vi "2012_12_29 Durability8 Main.vi"() -> ()   [LabVIEW 2011]
uses:
  MotorTypeDef.ctl
  <vilib>/DAQmx/write.llb/DAQmx Write (Counter Time 1Chan 1Samp).vi
  <vilib>/DAQmx/read.llb/DAQmx Read (Analog 1D Wfm NChan NSamp).vi
  <vilib>/Utility/TradDaqScaling.llb/Convert Thermistor Reading (waveform).vi
  <vilib>/DAQmx/miscellaneous.llb/DAQmx Fill In Error Info.vi
  <vilib>/measure/madcrms.llb/Averaged DC-RMS for N Chan.vi
  <vilib>/measure/madcrms.llb/Basic Averaged DC-RMS for 1 Chan.vi
  <vilib>/measure/matone.llb/Extract Single Tone Information 1 Chan.vi
  <vilib>/express/express arith-compare/Formula/XNode/ExpressFormulaBlockNode.xnode
  <vilib>/measure/NI_MAPro.lvlib
panel:
  out "for loop":i32
  out "Saving Data":bool
  in  "Coarse File Path":path=path "Durability/coarse.lvm"
  in  "Fine File Path":path=path "Durability/fine.lvm"
  out "Voltages":waveform(dbl)[](graph)
  out "Currents":waveform(dbl)[](graph)
  out "RMS Voltages 2":waveform(dbl)(graph)
  in  "Motor 8":T1 {"Efficiency" format="%#_3g%%"; "Supply Voltage (V)" format="%#_3f"; "Power Output (W)" format="%#_3g"; "Power Usage (W)" format="%#_3g"; "Torque (mNm)" format="%#_3g"; "RPM" scale=0.0..40000.0 scale format="%#.6p"}
  in  "Motor 7":T1 {"Efficiency" format="%#_3g%%"; "Supply Voltage (V)" format="%#_3f"; "Power Output (W)" format="%#_3g"; "Power Usage (W)" format="%#_3g"; "Torque (mNm)" format="%#_3g"; "RPM" scale=0.0..40000.0 scale format="%#.6p"}
  in  "Motor 6":T1 {"Efficiency" format="%#_3g%%"; "Supply Voltage (V)" format="%#_3f"; "Power Output (W)" format="%#_3g"; "Power Usage (W)" format="%#_3g"; "Torque (mNm)" format="%#_3g"; "RPM" scale=0.0..40000.0 scale format="%#.6p"}
  in  "Motor 5":T1 {"Efficiency" format="%#_3g%%"; "Supply Voltage (V)" format="%#_3f"; "Power Output (W)" format="%#_3g"; "Power Usage (W)" format="%#_3g"; "Torque (mNm)" format="%#_3g"; "RPM" scale=0.0..40000.0 scale format="%#.6p"}
  in  "Motor 4":T1 {"Efficiency" format="%#_3g%%"; "Supply Voltage (V)" format="%#_3f"; "Power Output (W)" format="%#_3g"; "Power Usage (W)" format="%#_3g"; "Torque (mNm)" format="%#_3g"; "RPM" scale=0.0..40000.0 scale format="%#.6p"}
  in  "Motor 3":T1 {"Efficiency" format="%#_3g%%"; "Supply Voltage (V)" format="%#_3f"; "Power Output (W)" format="%#_3g"; "Power Usage (W)" format="%#_3g"; "Torque (mNm)" format="%#_3g"; "RPM" scale=0.0..40000.0 scale format="%#.6p"}
  in  "Motor 2":T1 {"Efficiency" format="%#_3g%%"; "Supply Voltage (V)" format="%#_3f"; "Power Output (W)" format="%#_3g"; "Power Usage (W)" format="%#_3g"; "Torque (mNm)" format="%#_3g"; "RPM" scale=0.0..40000.0 scale format="%#.6p"}
  in  "Motor 1":T1 {"Efficiency" format="%#_3g%%"; "Supply Voltage (V)" format="%#_3f"; "Power Output (W)" format="%#_3g"; "Power Usage (W)" format="%#_3g"; "Torque (mNm)" format="%#_3g"; "RPM" scale=0.0..40000.0 scale format="%#.6p"}
  out "Motor Temp":dbl(slide) scale=90.0..110.0
  out "Tank Temp":dbl(slide) scale=90.0..110.0
  out "RMS Voltages":waveform(dbl)[](graph)
  out "RMS Currents":waveform(dbl)[](graph)
  in  "Temp Probe\nOn Motor":dbl=1.0
  out "loop time (ms)":u32
  in  "stop":bool
  in  "Unlock PWM":bool=TRUE
  in  "PWM 2":dbl(slide)=100.0 min=0.0 max=100.0 step=5.0 scale=0.0..100.0
  in  "PWM 1":dbl(slide) min=0.0 max=100.0 step=5.0 scale=0.0..100.0
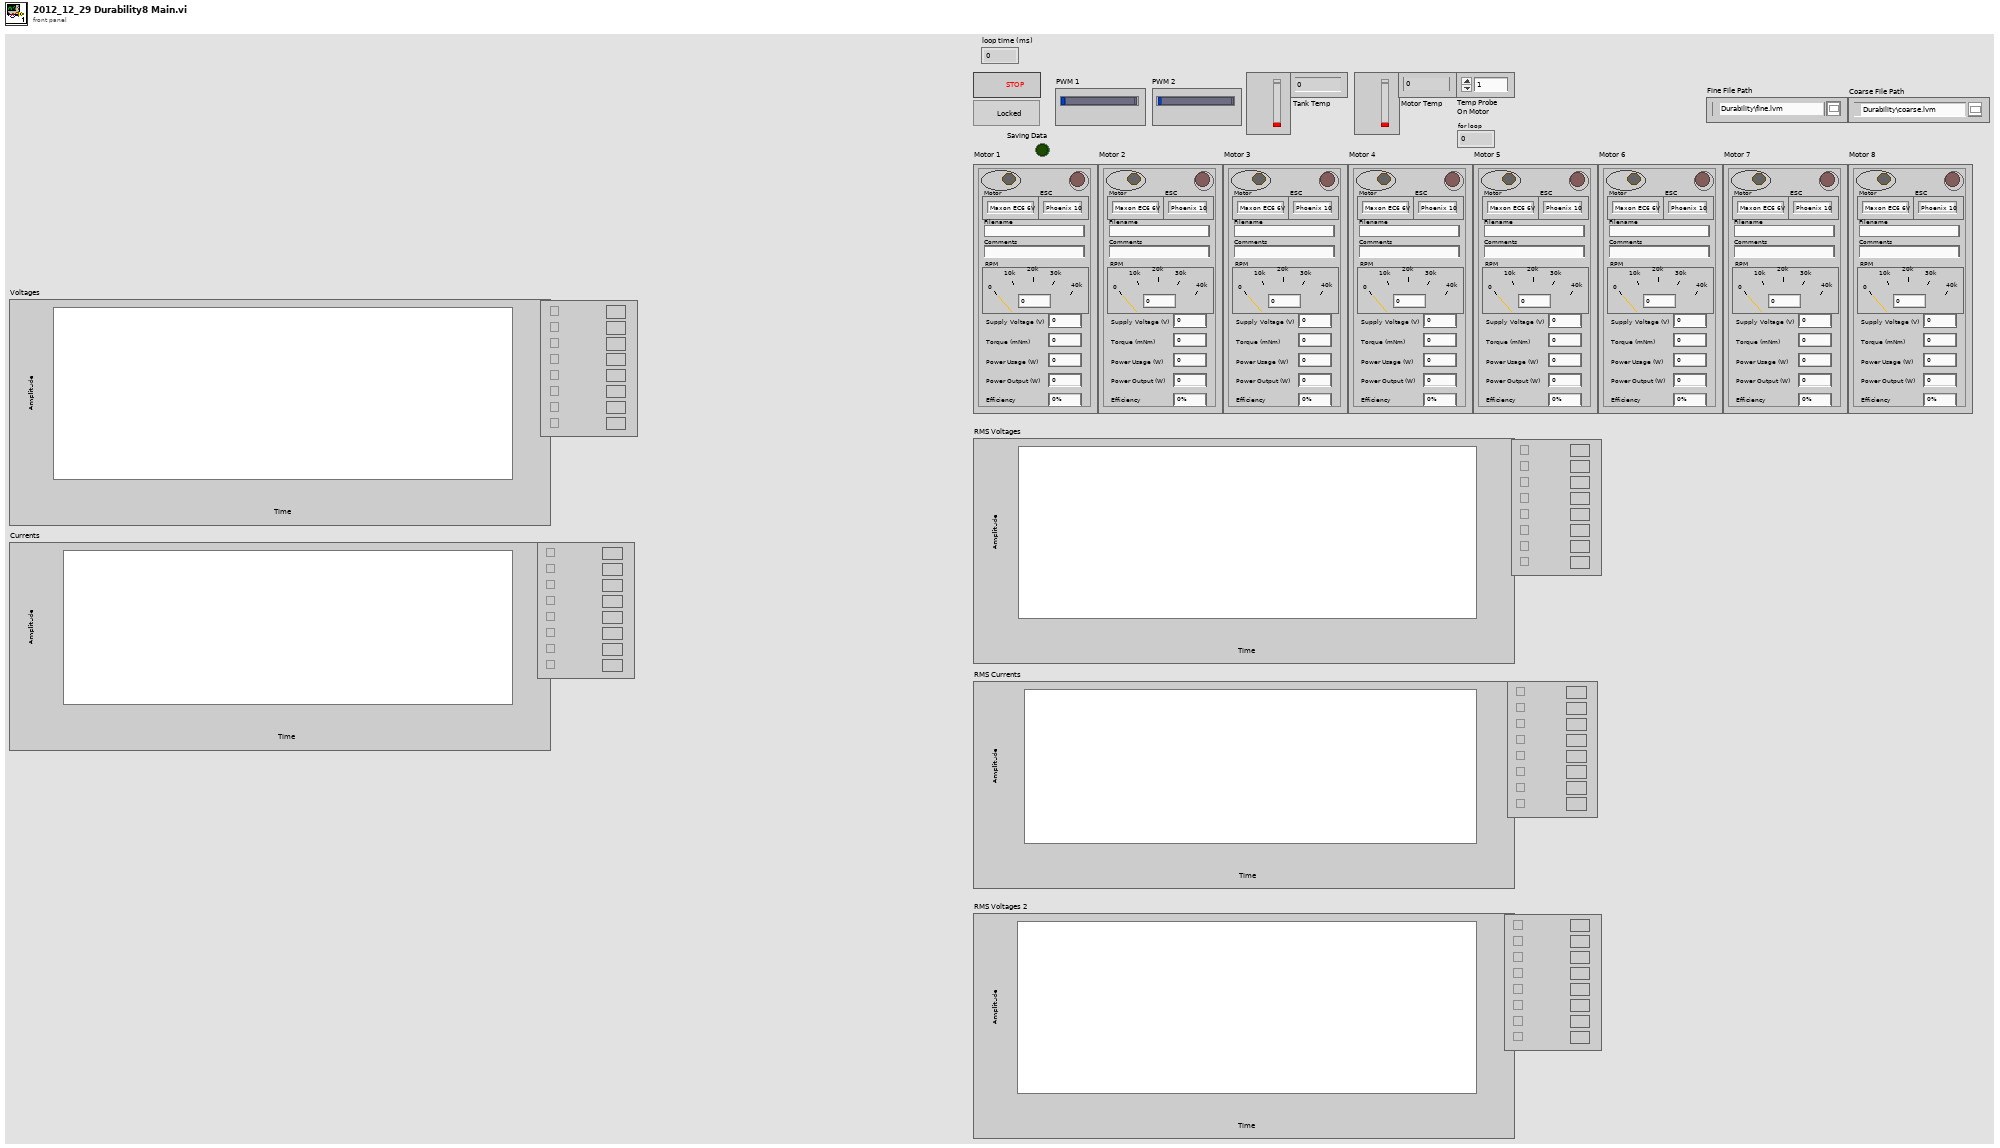
[diagram p1: front panel]
types:
  T1 = typedef "MotorTypeDef.ctl" = cluster{"Enabled":bool, "Fail":bool, "RPM":dbl, "Motor":enum16{"Maxon EC6 6V", "Maxon EC4 6V", "FH 0620 6V", "FH 0620 12V"}, "ESC":enum16{"Phoenix 10", "Maxon", "FH 1801"}, "Torque (mNm)":dbl, "Power Usage (W)":dbl, "Power Output (W)":dbl, "Supply Voltage (V)":dbl, "Efficiency":dbl, "Filename":string, "Comments":string}
  T2 = enum8{"Enabled", "Disabled", "Disabled and Grayed Out"}
  T3 = enum16{"Maxon EC6 6V", "Maxon EC4 6V", "FH 0620 6V", "FH 0620 12V"}
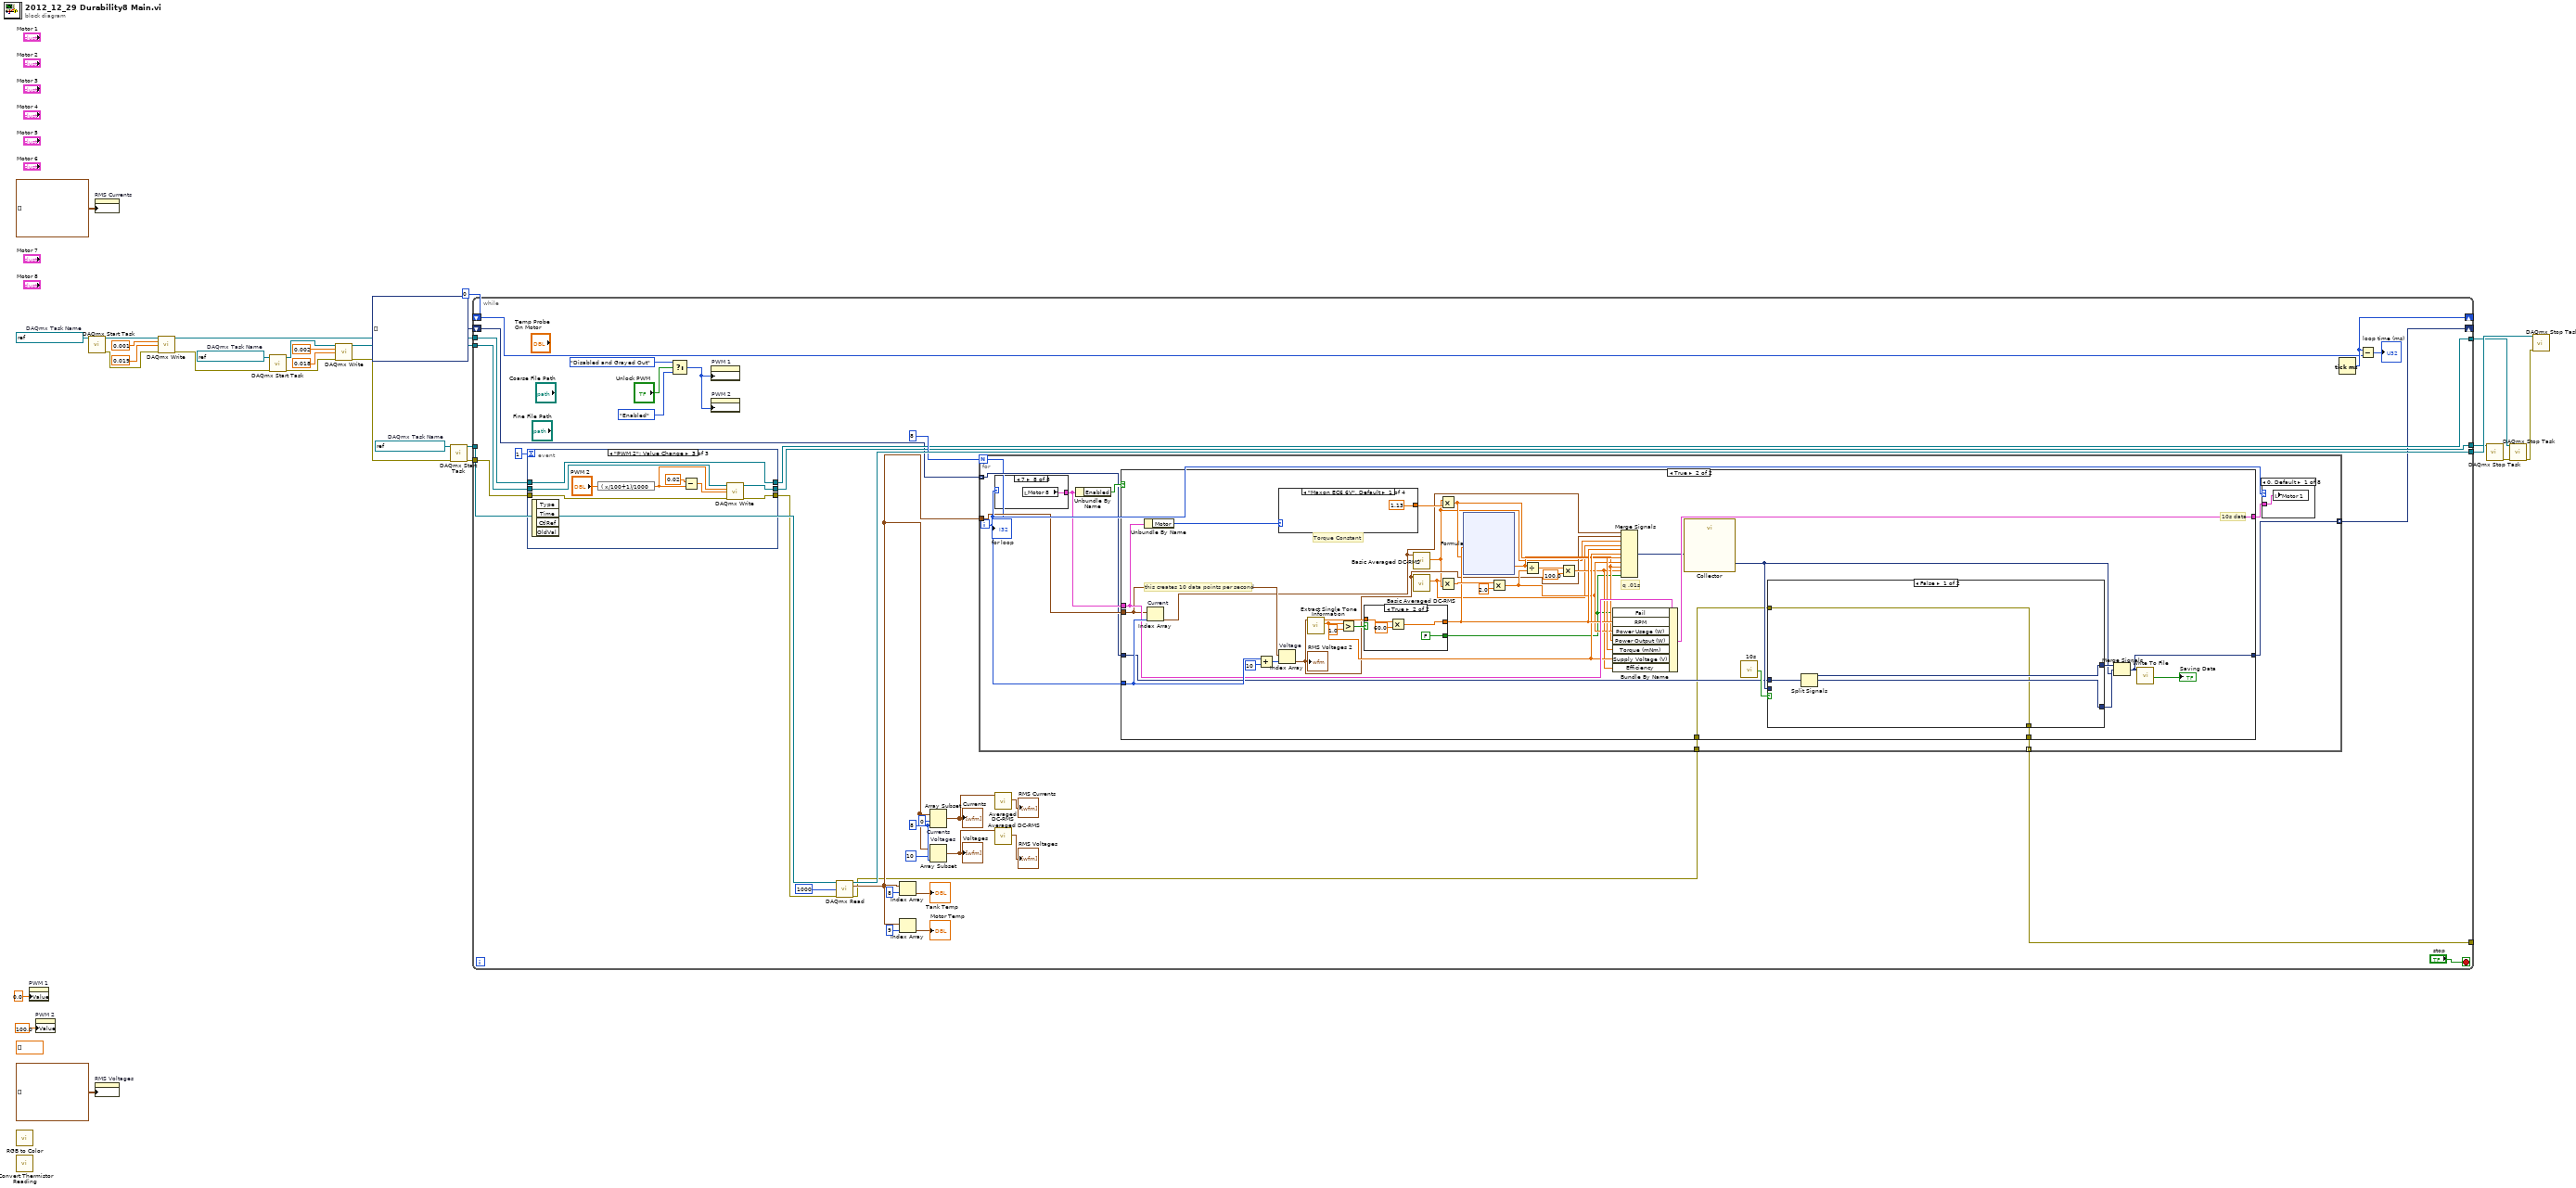
[diagram p0: block diagram]
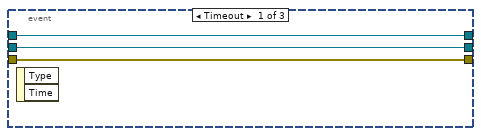
[diagram p2: hidden frame]
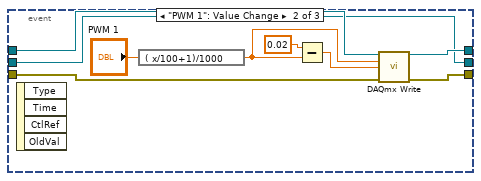
[diagram p3: hidden frame]
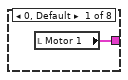
[diagram p4: hidden frame]
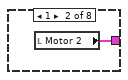
[diagram p5: hidden frame]
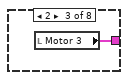
[diagram p6: hidden frame]
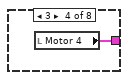
[diagram p7: hidden frame]
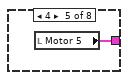
[diagram p8: hidden frame]
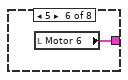
[diagram p9: hidden frame]
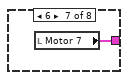
[diagram p10: hidden frame]
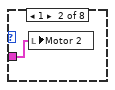
[diagram p11: hidden frame]
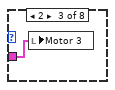
[diagram p12: hidden frame]
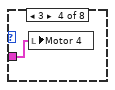
[diagram p13: hidden frame]
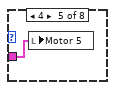
[diagram p14: hidden frame]
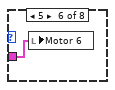
[diagram p15: hidden frame]
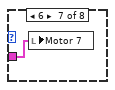
[diagram p16: hidden frame]
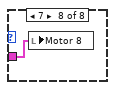
[diagram p17: hidden frame]
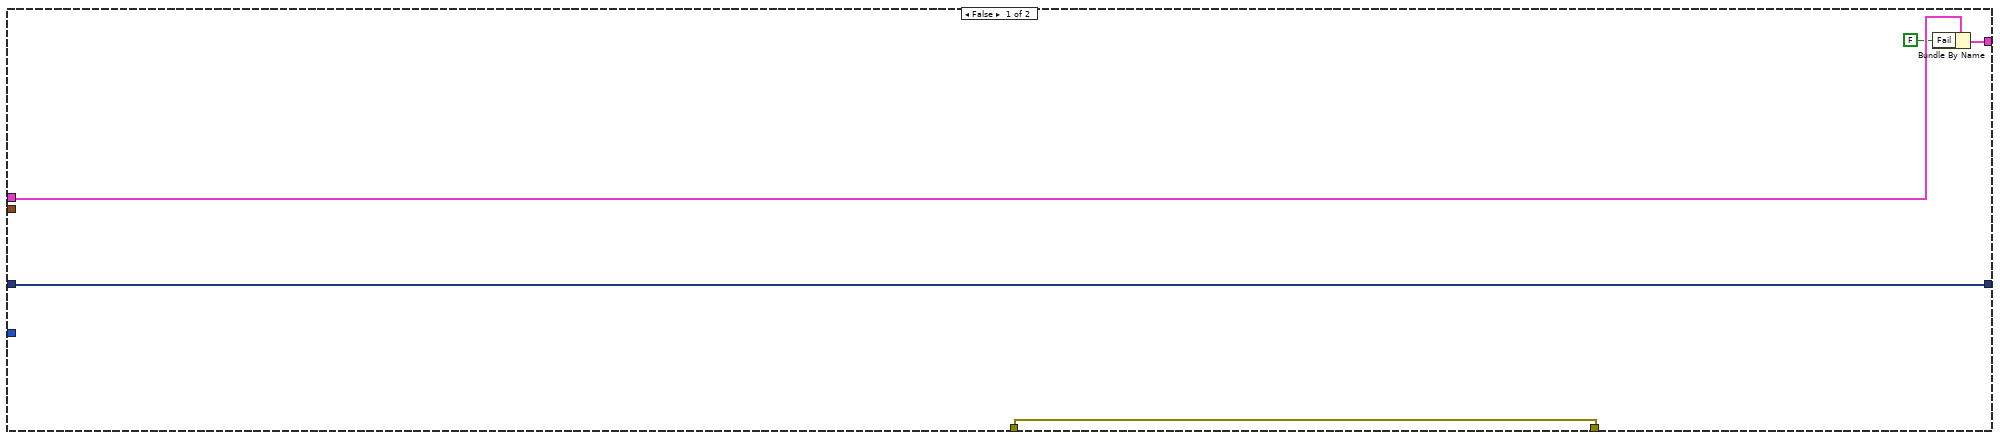
[diagram p18: hidden frame]
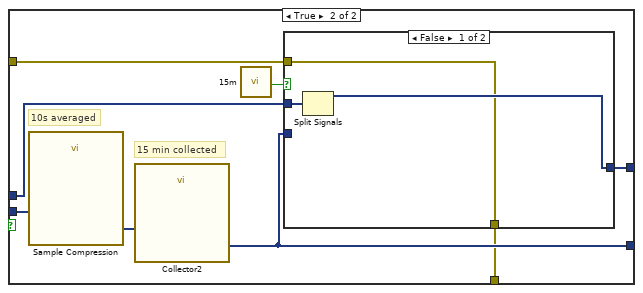
[diagram p19: hidden frame]
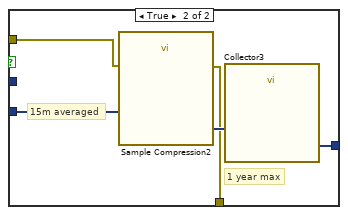
[diagram p20: hidden frame]
diagram:
  (unwired) dbl[] [] ("History Data")
  w23 = refnum<k21> "Durability8 PWM2"  # DAQmx Task Name
  w24 = refnum<k21> "Durability8 PWM1"  # DAQmx Task Name
  w28 = refnum<k21> "Durability8 Acquire"  # DAQmx Task Name
  n1 = call <vilib>:"RGB to Color.vi"() -> ()  [unwired: 3 in, 1 out]
  n2 = call-poly <vilib>:"Convert Thermistor Reading.vi"() -> ()  [unwired: 7 in, 1 out]
  n3 = property on="PWM 1" class="Slide (strict)"("Value"=0.0 ("PWM 1")) -> ()  [unwired: 2 in, 2 out]
  n4 = property on="PWM 2" class="Slide (strict)"("Value"=100.0 ("PWM 2")) -> ()  [unwired: 2 in, 2 out]
  n5 = call <vilib>:"DAQmx Start Task.vi"("task/channels in"=w24) -> ("task out"=w20:refnum<k21>, "error out"=w18:errorcluster)  [unwired: 13 in]
  n6 = property on="RMS Currents" class="WFChart (strict)"("History Data"=waveform(dbl)[][] []) -> ()  [unwired: 2 in, 2 out]
  n7 = property on="RMS Voltages" class="WFChart (strict)"("History Data"=waveform(dbl)[][] []) -> ()  [unwired: 2 in, 2 out]
  n8 = call-poly <vilib>:"DAQmx Write.vi"("task/channels in"=w20, "high time"=0.001 ("data"), "low time"=0.019 ("data"), "error in"=w18) -> ("task out"=w22:refnum<k21>, "error out"=w17:errorcluster)  [unwired: 9 in, 1 out]
  n9 = call <vilib>:"DAQmx Start Task.vi"("task/channels in"=w23, "error in"=w17) -> ("task out"=w19:refnum<k21>, "error out"=w16:errorcluster)  [unwired: 12 in]
  n10 = call-poly <vilib>:"DAQmx Write.vi"("task/channels in"=w19, "high time"=0.002 ("data"), "low time"=0.018 ("data"), "error in"=w16) -> ("task out"=w21:refnum<k21>, "error out"=w15:errorcluster)  [unwired: 9 in, 1 out]
  n11 = call <vilib>:"DAQmx Start Task.vi"("task/channels in"=w28, "error in"=w15) -> ("task out"=w27:refnum<k21>, "error out"=w25:errorcluster)  [unwired: 12 in]
  n12 = while {
    tunnel: w27 -> [w63]
    tunnel: [w62] -> w26
    tunnel: w25 -> [w39]
    tunnel: [w29] -> _
    shift-right: [w56] -> _
    shift-left: u32 0 ("millisecond timer value") -> [w55]
    tunnel: w22 -> [w41]
    tunnel: w21 -> [w40]
    tunnel: [w38] -> w14
    tunnel: [w37] -> w5
    shift-right: [w32] -> _
    shift-left: dynamicdata[] [] -> [w31]
    stop <- "stop" stop-if-true
    w51 = 8 ("length")
    n13 = event shown="[2] \"PWM 2\": Value Change" {
      selector: _ -> [_ _ _]
      dyn-events: _ -> [_ _ _]
      timeout: 1 -> [_ _ _]
      tunnel: w41 -> [w66 w71 w77]
      tunnel: w40 -> [w65 w69 w76]
      tunnel: [w66 w70 w77] -> w38
      tunnel: [w65 w69 w78] -> w37
      tunnel: [w64 w68 w79] -> w33
      tunnel: w39 -> [w64 w67 w80]
      event Timeout {
        n14 = event-data() -> ()  [unwired: 1 in, 2 out]
      }
      event "PWM 1": Value Change {
        n15 = event-data() -> ()  [unwired: 1 in, 4 out]
        n16 = expression code="( x/100+1)/1000"("PWM 1") -> (w72:dbl)
        n17 = Subtract(x=0.02 ("y"), y=w72) -> (x-y=w73:dbl)
        n18 = call-poly <vilib>:"DAQmx Write.vi"("task/channels in"=w71, "high time"=w72, "low time"=w73, "error in"=w67) -> ("task out"=w70:refnum<k21>, "error out"=w68:errorcluster)  [unwired: 9 in, 1 out]
      }
      event "PWM 2": Value Change {
        n19 = event-data() -> ()  [unwired: 1 in, 4 out]
        n20 = expression code="( x/100+1)/1000"("PWM 2") -> (w84:dbl)
        n21 = Subtract(x=0.02, y=w84) -> (x-y=w82:dbl)
        n22 = call-poly <vilib>:"DAQmx Write.vi"("task/channels in"=w76, "high time"=w84, "low time"=w82, "error in"=w80) -> ("task out"=w78:refnum<k21>, "error out"=w79:errorcluster)  [unwired: 9 in, 1 out]
      }
    }
    n23 = Select(t=T2."Disabled and Grayed Out" ("Disabled"), s="Unlock PWM", f=T2."Enabled" ("Disabled")) -> (s? t:f=w60:T2)
    n24 = property on="PWM 1" class="Slide (strict)"("DisabledEnum"=w60) -> ()  [unwired: 2 in, 2 out]
    n25 = property on="PWM 2" class="Slide (strict)"("DisabledEnum"=w60) -> ()  [unwired: 2 in, 2 out]
    n26 = call-poly <vilib>:"DAQmx Read.vi"("task/channels in"=w63, "number of samples per channel"=1000, "error in"=w33) -> ("task out"=w62:refnum<k21>, "data"=w43:waveform(dbl)[], "error out"=w30:errorcluster)  [unwired: 10 in]
    n27 = Index Array(array=w43, index=8) -> (element=→"Tank Temp":waveform(dbl))
    n28 = Index Array(array=w43, index=9) -> (element=→"Motor Temp":waveform(dbl))
    n29 = Array Subset "Currents"(array=w43, index=0, length=w51) -> (w35:waveform(dbl)[])
    "Currents" <- w35
    n30 = Array Subset "Voltages"(array=w43, index=10 ("length"), length=w51) -> (w34:waveform(dbl)[])
    "Voltages" <- w34
    n31 = for {
      N: 8 -> [w85]
      tunnel: w43 -> [w90]
      tunnel: [w89] -> w32 mode=indexing
      tunnel: w31 -> [w88] mode=indexing
      tunnel: w30 -> [w87]
      tunnel: [w86] -> w29 mode=indexing
      i -> [w93]
      n32 = case shown="7" w93 {
        tunnel: [w95 w96 w97 w98 w99 w100 w101 w102] -> w92
        frame 0, Default {
          n33 = local read "Motor 1"() -> (w95:T1)
        }
        frame 1 {
          n34 = local read "Motor 2"() -> (w96:T1)
        }
        frame 2 {
          n35 = local read "Motor 3"() -> (w97:T1)
        }
        frame 3 {
          n36 = local read "Motor 4"() -> (w98:T1)
        }
        frame 4 {
          n37 = local read "Motor 5"() -> (w99:T1)
        }
        frame 5 {
          n38 = local read "Motor 6"() -> (w100:T1)
        }
        frame 6 {
          n39 = local read "Motor 7"() -> (w101:T1)
        }
        frame 7 {
          n40 = local read "Motor 8"() -> (w102:T1)
        }
      }
      n41 = Unbundle By Name(w92) -> ("Enabled"=w94:bool)
      n42 = case shown="True" w94 {
        tunnel: w93 -> [_ w148]
        tunnel: w92 -> [w115 w143]
        tunnel: [w114 w142] -> w91
        tunnel: w90 -> [_ w130]
        tunnel: [w112 w119] -> w89
        tunnel: w88 -> [w112 w120]
        tunnel: w87 -> [w111 w117]
        tunnel: [w111 w116] -> w86
        frame False {
          n43 = Bundle By Name(cluster=w115, "Fail"=FALSE) -> (w114:T1)
        }
        frame True {
          # "10s data"
          # "q .01s"
          # "this creates 10 data points per second"
          # "Torque Constant"
          n44 = Unbundle By Name(w143) -> ("Motor"=w145:T3)
          n45 = Index Array "Current"(array=w130, index=w148) -> (element=w129:waveform(dbl))
          n46 = Add(x=w148, y=10) -> (x+y=w147:i32)
          n47 = case shown="\"Maxon EC6 6V\", Default" w145 {
            tunnel: [1.13 1.84 1.13 2.91] -> w144
            frame "Maxon EC6 6V", Default {
            }
            frame "Maxon EC4 6V" {
            }
            frame "FH 0620 6V" {
            }
            frame "FH 0620 12V" {
            }
          }
          n48 = Index Array "Voltage"(array=w130, index=w147) -> (element=w128:waveform(dbl))
          "RMS Voltages 2" <- w128
          n49 = call-poly <vilib>:"Extract Single Tone Information.vi"("time signal in"=w128) -> ("detected amplitude"=w136:dbl, "detected frequency"=w146:dbl)  [unwired: 5 in, 4 out]
          n50 = Greater?(x=w136, y=1.0) -> (0:w151:bool)
          n51 = case shown="True" w151 {
            tunnel: [0.0 ("y") w191] -> w137
            tunnel: w146 -> [_ w189]
            tunnel: [TRUE FALSE] -> w131
            frame False {
            }
            frame True {
              n52 = Multiply(x=w189, y=60.0) -> (x*y=w191:dbl)
            }
          }
          n53 = call-poly <vilib>:"Basic Averaged DC-RMS.vi"("signal in"=w129) -> ("RMS value"=w127:dbl)  [unwired: 7 in, 3 out]
          n54 = call-poly <vilib>:"Basic Averaged DC-RMS.vi"("signal in"=w128) -> ("RMS value"=w126:dbl)  [unwired: 7 in, 3 out]
          n55 = Multiply(x=w127, y=w144) -> (x*y=w135:dbl)
          n56 = Multiply(x=w126, y=w127) -> (x*y=w141:dbl)
          n57 = xnode "Formula"("RPM"=w137, "Torque"=w135) -> ("Result"=w133:dbl)  [unwired: 1 in, 1 out]
          n58 = Multiply(x=w141, y=2.0) -> (x*y=w134:dbl)
          n59 = Divide(x=w133, y=w134) -> (x/y=w139:dbl)
          n60 = Multiply(x=w139, y=100.0) -> (x*y=w132:dbl)
          n61 = Bundle By Name(cluster=w143, "Fail"=w131, "RPM"=w137, "Power Usage (W)"=w134, "Power Output (W)"=w133, "Torque (mNm)"=w135, "Supply Voltage (V)"=w136, "Efficiency"=w132) -> (w142:T1)
          n62 = Merge Signals(w129, w128, w127, w126, w137, w136, w135, w134, w133, w132, w131) -> (w125:dynamicdata)
          n63 = call "Collector"("Signals"=w125) -> ("Collected Signals"=w121:dynamicdata)  [unwired: 9 in, 1 out]
          n64 = call "10s"() -> ("Time has Elapsed"=w124:bool)  [unwired: 12 in, 7 out]
          n65 = case shown="False" w124 {
            tunnel: w121 -> [_ w163]
            tunnel: [w154 w160] -> w123
            tunnel: [w153 w159] -> w122
            tunnel: w120 -> [w155 w158]
            tunnel: w117 -> [w152 w157]
            tunnel: [w152 w156] -> w116
            frame False {
              n66 = Split Signals(w155) -> (w154:dynamicdata, w153:dynamicdata)  [unwired: 3 in, 1 out]
            }
            frame True {
              # "15 min collected"
              # "10s averaged"
              n67 = call "Sample Compression"("Signals"=w163) -> ("Mean"=w162:dynamicdata)  [unwired: 8 in, 2 out]
              n68 = call "Collector2"("Signals"=w162) -> ("Collected Signals"=w159:dynamicdata)  [unwired: 9 in, 1 out]
              n69 = call "15m"() -> ("Time has Elapsed"=w161:bool)  [unwired: 12 in, 7 out]
              n70 = case shown="False" w161 {
                tunnel: w159 -> [_ w171]
                tunnel: [w165 w169] -> w160
                tunnel: w158 -> [w166 _]
                tunnel: w157 -> [w164 w168]
                tunnel: [w164 w167] -> w156
                frame False {
                  n71 = Split Signals(w166) -> (w165:dynamicdata)  [unwired: 3 in, 2 out]
                }
                frame True {
                  # "1 year max"
                  # "15m averaged"
                  n72 = call "Sample Compression2"("error in (no error)"=w168, "Signals"=w171) -> ("error out"=w167:errorcluster, "Mean"=w170:dynamicdata)  [unwired: 7 in, 1 out]
                  n73 = call "Collector3"("Signals"=w170) -> ("Collected Signals"=w169:dynamicdata)  [unwired: 9 in, 1 out]
                }
              }
            }
          }
          n74 = Merge Signals(w123, w122, w121) -> (w119:dynamicdata)
          n75 = call "Write To File"("Signals"=w119) -> ("Saving Data"=→"Saving Data":bool)  [unwired: 16 in, 2 out]
        }
      }
      n76 = case shown="0, Default" w93 {
        tunnel: w91 -> [w103 w104 w105 w106 w107 w108 w109 w110]
        frame 0, Default {
          n77 = local write "Motor 1"(w103) -> ()
        }
        frame 1 {
          n78 = local write "Motor 2"(w104) -> ()
        }
        frame 2 {
          n79 = local write "Motor 3"(w105) -> ()
        }
        frame 3 {
          n80 = local write "Motor 4"(w106) -> ()
        }
        frame 4 {
          n81 = local write "Motor 5"(w107) -> ()
        }
        frame 5 {
          n82 = local write "Motor 6"(w108) -> ()
        }
        frame 6 {
          n83 = local write "Motor 7"(w109) -> ()
        }
        frame 7 {
          n84 = local write "Motor 8"(w110) -> ()
        }
      }
      "for loop" <- w85
    }
    n85 = call-poly <vilib>:"Averaged DC-RMS.vi"("signals in"=w35) -> ("RMS value waveforms"=→"RMS Currents":waveform(dbl)[])  [unwired: 6 in, 4 out]
    n86 = call-poly <vilib>:"Averaged DC-RMS.vi"("signals in"=w34) -> ("RMS value waveforms"=→"RMS Voltages":waveform(dbl)[])  [unwired: 6 in, 4 out]
    n87 = Tick Count (ms)() -> (millisecond timer value=w56:u32)
    n88 = Subtract(x=w56, y=w55) -> (x-y=→"loop time (ms)":u32)
  }
  n89 = call <vilib>:"DAQmx Stop Task.vi"("task/channels in"=w5) -> ("error out"=w13:errorcluster)  [unwired: 13 in, 1 out]
  n90 = call <vilib>:"DAQmx Stop Task.vi"("task/channels in"=w14, "error in"=w13) -> ("error out"=w12:errorcluster)  [unwired: 12 in, 1 out]
  n91 = call <vilib>:"DAQmx Stop Task.vi"("task/channels in"=w26, "error in"=w12) -> ()  [unwired: 12 in, 2 out]
